vi "Window Max.vi"(8 "error in (no error)":errorcluster, 11 "last level":i32=2) -> (0 "error out":errorcluster)   [LabVIEW 2020]
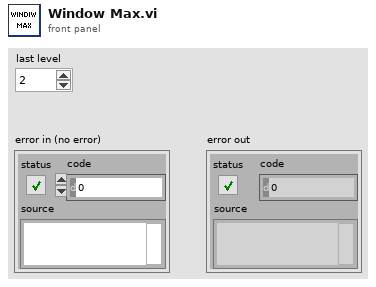
[diagram p1: front panel]
types:
  T1 = enum32{"Invalid", "Standard", "Closed", "Hidden", "Minimized", "Maximized"}
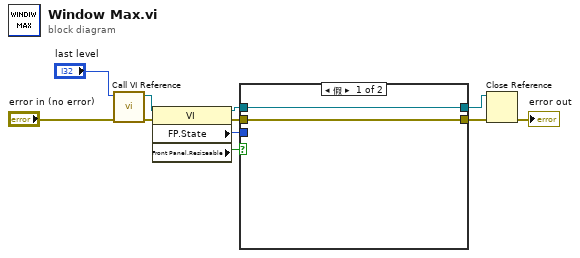
[diagram p0: block diagram]
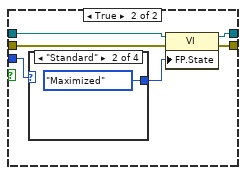
[diagram p2: hidden frame]
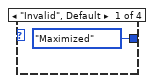
[diagram p3: hidden frame]
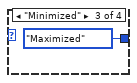
[diagram p4: hidden frame]
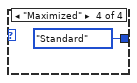
[diagram p5: hidden frame]
diagram:
  n1 = call "Call VI Reference.vi"("error in"="error in (no error)", "last level"="last level") -> ("error out"=w5:errorcluster, "vi reference out"=w6:refnum<vi>)  [unwired: 8 in]
  n2 = property class="VI"(reference=w6, error in=w5) -> (reference out=w10:refnum<vi>, error out=w9:errorcluster, "FP.State"=w11:T1, "Front Panel.Resizeable"=w1:bool)
  n3 = case shown="假" w1 {
    tunnel: w11 -> [_ w19]
    tunnel: w10 -> [w13 w18]
    tunnel: w9 -> [w12 w17]
    tunnel: [w13 w16] -> w8
    tunnel: [w12 w15] -> w7
    frame False {
    }
    frame True {
      n4 = case shown="\"Standard\"" w19 {
        tunnel: [T1."Maximized" ("前面板窗口:状态") T1."Maximized" ("前面板窗口:状态") T1."Maximized" ("前面板窗口:状态") T1."Standard" ("前面板窗口:状态")] -> w14
        frame "Invalid", Default {
        }
        frame "Standard" {
        }
        frame "Minimized" {
        }
        frame "Maximized" {
        }
      }
      n5 = property class="VI"(reference=w18, error in=w17, "FP.State"=w14) -> (reference out=w16:refnum<vi>, error out=w15:errorcluster)
    }
  }
  n6 = Close Reference(reference=w8, error in (no error)=w7) -> (error out=→"error out":errorcluster)
